vi "AG34980A_Switch.vi"(0 "VISA resource name":refnum<visa-resource-name>, 1 "Channel List":string, 5 "Open/Close (0:Close)":enum16{"Close", "Open"}(ring), 7 "Close Exclusive (F:Normal)":bool, 11 "error in (no error)":errorcluster, 12 "Set/Check (F:Set)":bool) -> (4 "VISA resource name out":refnum<visa-resource-name>, 6 "Channel State?":string, 15 "error out":errorcluster)   [LabVIEW 2022 SP3]
doc: "This VI lets you open/close a list of channels in the various switching modules."
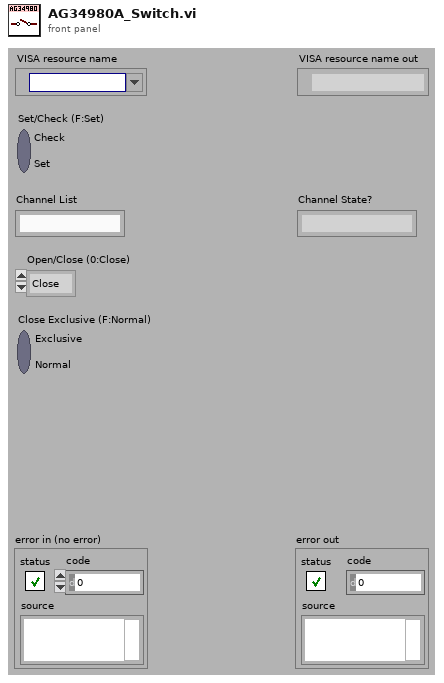
[diagram p1: front panel]
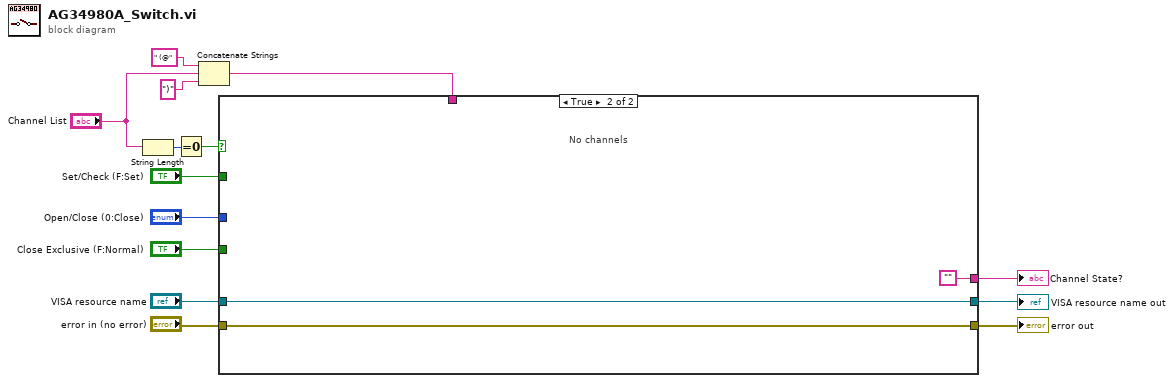
[diagram p0: block diagram]
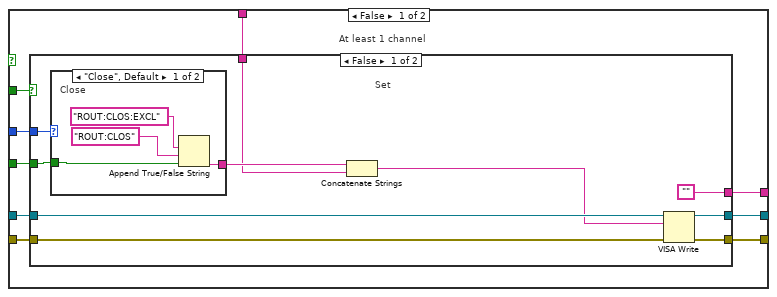
[diagram p2: hidden frame]
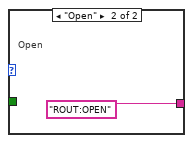
[diagram p3: hidden frame]
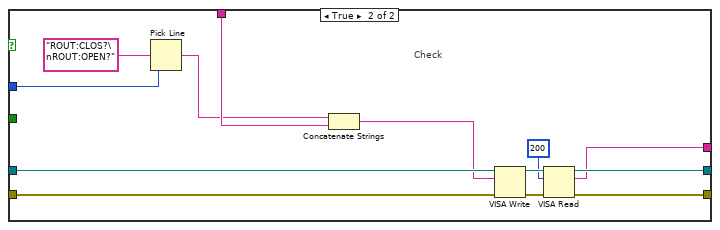
[diagram p4: hidden frame]
diagram:
  n1 = String Length(string="Channel List") -> (length=w7:i32)
  n2 = Equal To 0?(x=w7) -> (x = 0?=w9:bool)
  n3 = Concatenate Strings(" (@", "Channel List", ")") -> (w8:string)
  n4 = case shown="True" w9 {
    tunnel: [w23 ""] -> w10
    tunnel: [w22 w53] -> w2
    tunnel: [w21 w54] -> w1
    tunnel: "error in (no error)" -> [w20 w53]
    tunnel: "VISA resource name" -> [w19 w54]
    tunnel: w8 -> [w18 _]
    tunnel: "Close Exclusive (F:Normal)" -> [w17 _]
    tunnel: "Open/Close (0:Close)" -> [w16 _]
    tunnel: "Set/Check (F:Set)" -> [w15 _]
    frame False {
      # "At least 1 channel"
      n5 = case shown="False" w15 {
        tunnel: w16 -> [w33 w39]
        tunnel: w17 -> [w32 _]
        tunnel: w18 -> [w25 w51]
        tunnel: w19 -> [w30 w45]
        tunnel: w20 -> [w29 w44]
        tunnel: [w28 w50] -> w21
        tunnel: [w27 w48] -> w22
        tunnel: ["" w49] -> w23
        frame False {
          # "Set"
          n6 = case shown="\"Close\", Default" w33 {
            tunnel: w32 -> [w37 _]
            tunnel: [w34 "ROUT:OPEN"] -> w31
            frame "Close", Default {
              # "Close"
              n7 = Append True/False String(1:w37, 2:"ROUT:CLOS", 3:"ROUT:CLOS:EXCL") -> (0:w34:string)  [unwired: 1 in]
            }
            frame "Open" {
              # "Open"
            }
          }
          n8 = Concatenate Strings(w31, w25) -> (w24:string)
          n9 = VISA Write(VISA resource name=w30, write buffer=w24, error in (no error)=w29) -> (VISA resource name out=w28:refnum<visa-resource-name>, error out=w27:errorcluster)  [unwired: 1 out]
        }
        frame True {
          # "Check"
          n10 = Pick Line(multi-line string="ROUT:CLOS?\nROUT:OPEN?", line index=w39) -> (output string=w41:string)  [unwired: 1 in]
          n11 = Concatenate Strings(w41, w51) -> (w43:string)
          n12 = VISA Write(VISA resource name=w45, write buffer=w43, error in (no error)=w44) -> (VISA resource name out=w47:refnum<visa-resource-name>, error out=w46:errorcluster)  [unwired: 1 out]
          n13 = VISA Read(VISA resource name=w47, byte count=u32 200 ("byte count (0)"), error in (no error)=w46) -> (VISA resource name out=w50:refnum<visa-resource-name>, read buffer=w49:string, error out=w48:errorcluster)  [unwired: 1 out]
        }
      }
    }
    frame True {
      # "No channels"
    }
  }
  "Channel State?" <- w10
  "VISA resource name out" <- w1
  "error out" <- w2
